vi "Keithley 2182 Edit Settings.vi"(8 "error in":errorcluster, 11 "Instrument parameters in":T1) -> (0 "error out":errorcluster, 3 "Instrument parameters out":T1)   [LabVIEW 2025]
doc: "Sets a reference for the specified measurement and reads a single Rel'd Measurement."
uses:
  Keithley 2182.lvlib
panel:
  in  "Check measurement":bool
  in  "Boolean 2":bool
  in  "Boolean":bool
  out "error out":errorcluster
  in  "stop":bool
  in  "Voltage Resolution (8)":i32=8
  in  "Range Value (0)":dbl=10.0
  in  "Auto Range (T: Enable)":bool=TRUE
  out "Measurement":dbl
  out "Measurement Metadata":T2
  in  "Measurement (0: Voltage Channel 1)":i32(ring) items=["Voltage Channel 1", "Voltage Channel 2", "Temperature Channel 1", "Temperature Channel 2"]
  in  "Integration Rate Units (0: Line Cycles)":i32(ring) items=["Line Cycles", "Seconds"]
  in  "Integration Rate (5)":dbl=5.0
  # "Settings for Keithley 2182 ..."
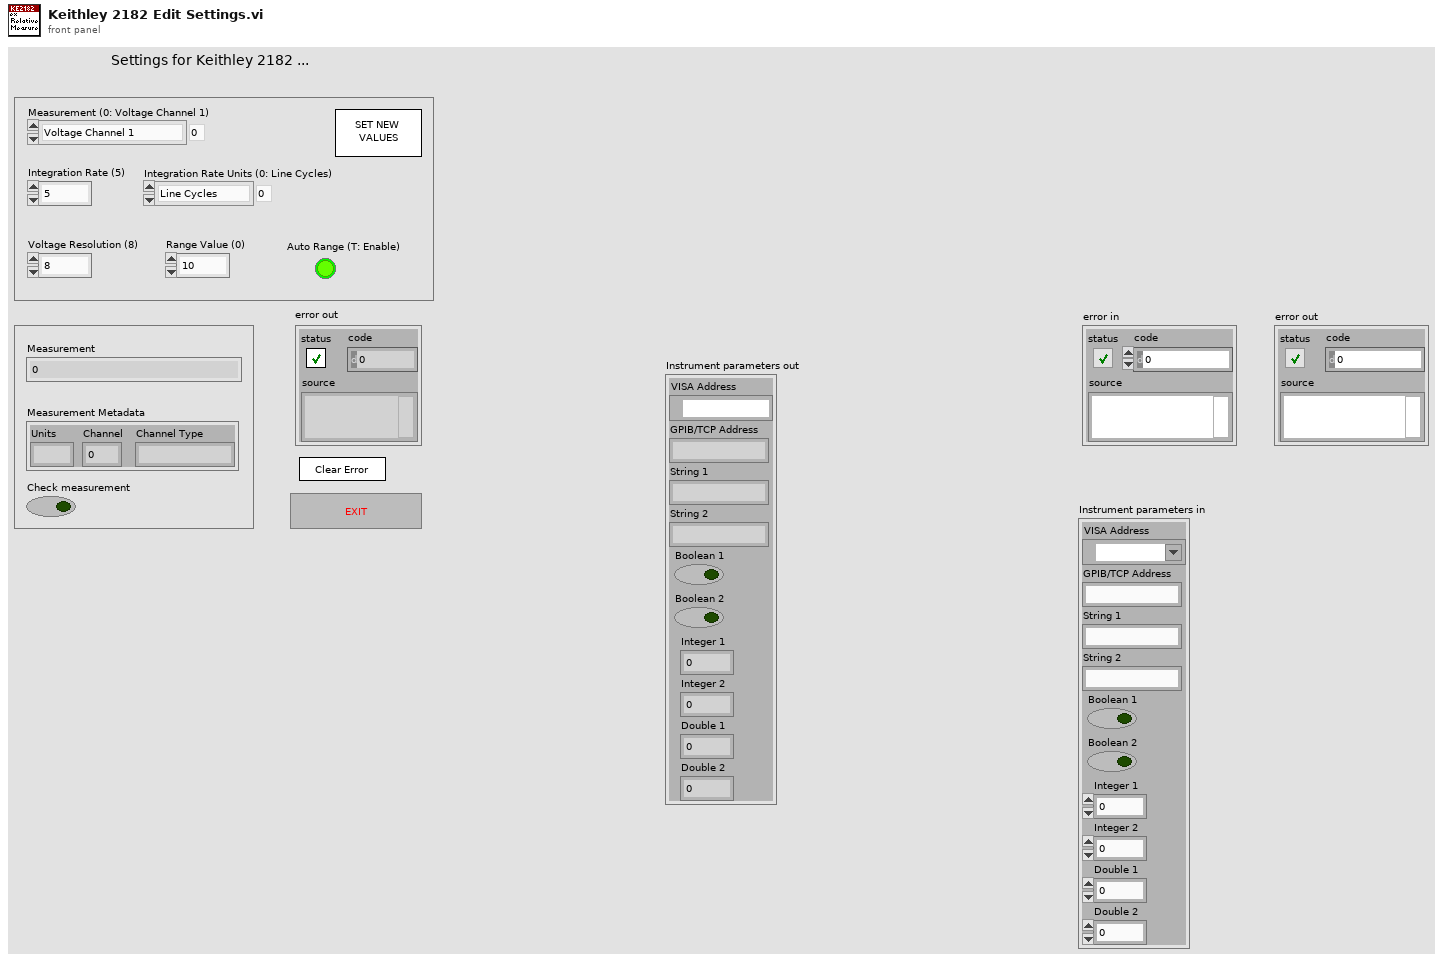
[diagram p1: front panel]
types:
  T1 = cluster{"VISA Address":refnum<visa-resource-name>, "GPIB/TCP Address":string, "String 1":string, "String 2":string, "Boolean 1":bool, "Boolean 2":bool, "Integer 1":i32, "Integer 2":i32, "Double 1":dbl, "Double 2":dbl}
  T2 = cluster{"Units":string, "Channel":i32, "Channel Type":string}
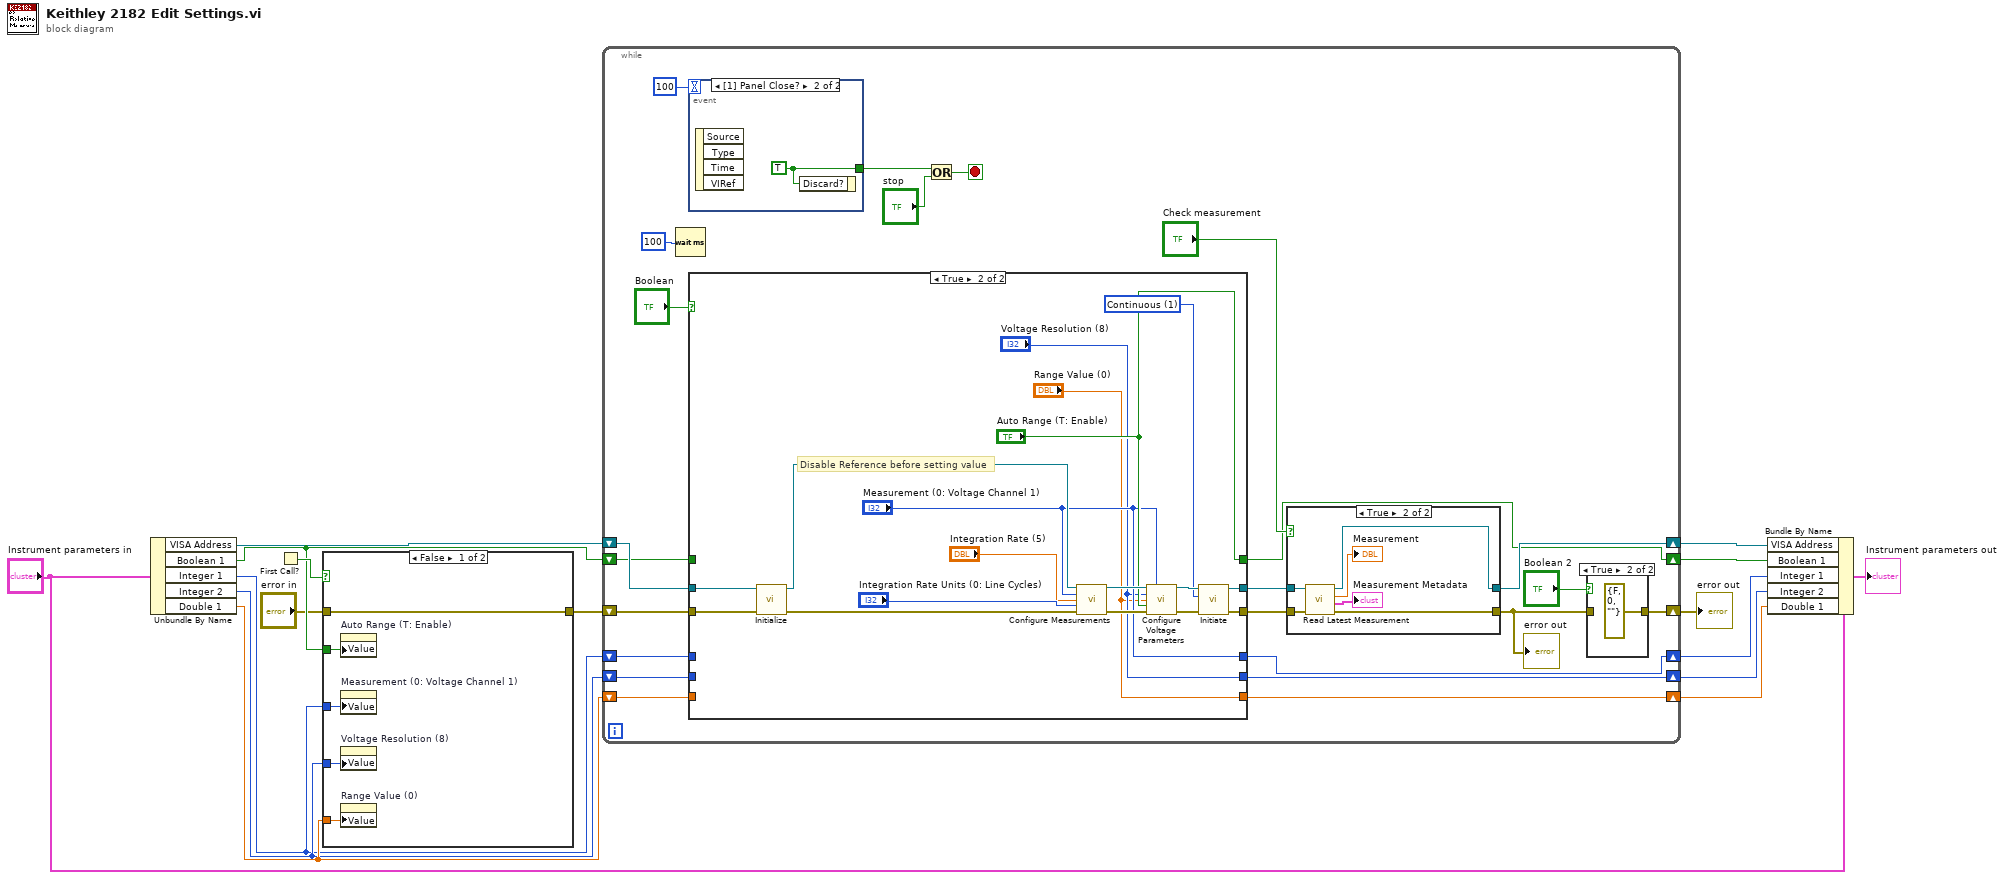
[diagram p0: block diagram]
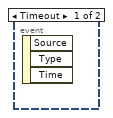
[diagram p6: hidden frame]
diagram:
  n1 = Unbundle By Name("Instrument parameters in") -> ("VISA Address"=w15:refnum<visa-resource-name>, "Boolean 1"=w4:bool, "Integer 1"=w3:i32, "Integer 2"=w5:i32, "Double 1"=w6:dbl)
  n2 = First Call?() -> (First Call?: T/F=w7:bool)
  n3 = case shown="False" w7 {
    tunnel: w6 -> [w21 _]
    tunnel: w5 -> [w20 _]
    tunnel: w4 -> [w18 _]
    tunnel: w3 -> [w19 _]
    tunnel: [w17 w22] -> w2
    tunnel: "error in" -> [w17 w22]
    frame False {
      n4 = property on="Auto Range (T: Enable)" class="Bool (strict)"("Value"=w18) -> ()  [unwired: 2 in, 2 out]
      n5 = property on="Measurement (0: Voltage Channel 1)" class="Ring (strict)"("Value"=w19) -> ()  [unwired: 2 in, 2 out]
      n6 = property on="Voltage Resolution (8)" class="DigNum (strict)"("Value"=w20) -> ()  [unwired: 2 in, 2 out]
      n7 = property on="Range Value (0)" class="DigNum (strict)"("Value"=w21) -> ()  [unwired: 2 in, 2 out]
    }
    frame True {
    }
  }
  n8 = while {
    shift-right: [w41] -> w13
    shift-left: w15 -> [w42]
    shift-right: [w34] -> w16
    shift-left: w2 -> [w40]
    shift-right: [w30] -> w11
    shift-left: w4 -> [w29]
    shift-right: [w28] -> w10
    shift-left: w3 -> [w27]
    shift-right: [w26] -> w9
    shift-left: w5 -> [w25]
    shift-right: [w23] -> w8
    shift-left: w6 -> [w24]
    stop <- w37 stop-if-true
    n9 = Wait (ms)(milliseconds to wait=u32 100) -> ()  [unwired: 1 out]
    n10 = event shown="[1] Panel Close?" {
      selector: _ -> [_ _]
      dyn-events: _ -> [_ _]
      timeout: 100 -> [_ _]
      tunnel: [_ w79] -> w39
      event Timeout {
        n11 = event-data() -> ()  [unwired: 1 in, 3 out]
      }
      event Panel Close? {
        w79 = TRUE ("Discard?")
        n12 = event-data() -> ()  [unwired: 1 in, 4 out]
        n13 = event-data("Discard?"=w79) -> ()  [unwired: 1 in, 1 out]
      }
    }
    n14 = case shown="True" "Boolean" {
      tunnel: [w60 w70] -> w45
      tunnel: [w61 w69] -> w44
      tunnel: w42 -> [w61 w67]
      tunnel: w40 -> [w60 w66]
      tunnel: [w59 "Auto Range (T: Enable)"] -> w30
      tunnel: w29 -> [w59 _]
      tunnel: [w58 "Measurement (0: Voltage Channel 1)"] -> w28
      tunnel: w27 -> [w58 _]
      tunnel: [w57 "Voltage Resolution (8)"] -> w26
      tunnel: w25 -> [w57 _]
      tunnel: [w56 "Range Value (0)"] -> w23
      tunnel: w24 -> [w56 _]
      frame False {
      }
      frame True {
        w68 = 1 items=["Immediate", "Continuous"] ("Initiate Type (0: Immediate)")
        # "Disable Reference before setting value"
        n15 = call "Initialize.vi"("error in (no error)"=w66, "VISA resource name"=w67) -> ("error out"=w78:errorcluster, "VISA resource name out"=w77:refnum<visa-resource-name>)  [unwired: 8 in]
        n16 = call "Configure Measurements.vi"("VISA resource name"=w77, "Measurement (0: Voltage Channel 1)"="Measurement (0: Voltage Channel 1)", "Integration Rate (5)"="Integration Rate (5)", "Integration Rate Units (0: Line Cycles)"="Integration Rate Units (0: Line Cycles)", "error in (no error)"=w78) -> ("VISA resource name out"=w73:refnum<visa-resource-name>, "error out"=w74:errorcluster)  [unwired: 9 in]
        n17 = call "Configure Voltage Parameters.vi"("VISA resource name"=w73, "Measurement (1: Voltage Channel 1)"="Measurement (0: Voltage Channel 1)", "Voltage Resolution (8)"="Voltage Resolution (8)", "Range Value (12)"="Range Value (0)", "Autorange (T: Enable)"="Auto Range (T: Enable)", "error in (no error)"=w74) -> ("VISA resource name out"=w71:refnum<visa-resource-name>, "error out"=w72:errorcluster)  [unwired: 8 in]
        n18 = call "Initiate.vi"("error in (no error)"=w72, "Initiate Type (0: Immediate)"=w68, "VISA resource name"=w71) -> ("error out"=w70:errorcluster, "VISA resource name out"=w69:refnum<visa-resource-name>)  [unwired: 7 in]
      }
    }
    n19 = Or(x=w39, y="stop") -> (x .or. y?=w37:bool)
    n20 = case shown="True" "Check measurement" {
      tunnel: w45 -> [w46 w53]
      tunnel: w44 -> [w47 w52]
      tunnel: [w47 w51] -> w41
      tunnel: [w46 w50] -> w33
      frame False {
      }
      frame True {
        n21 = call "Read Latest Measurement.vi"("error in (no error)"=w53, "VISA resource name"=w52) -> ("error out"=w50:errorcluster, "Measurement Metadata"=→"Measurement Metadata":T2, "Measurement"=→"Measurement":dbl, "VISA resource name out"=w51:refnum<visa-resource-name>)  [unwired: 6 in]
      }
    }
    "error out" <- w33
    n22 = case shown="True" "Boolean 2" {
      tunnel: [w54 errorcluster {"status"=FALSE, "code"=0, "source"=""} ("error out")] -> w34
      tunnel: w33 -> [w54 _]
      frame False {
      }
      frame True {
      }
    }
  }
  "error out" <- w16
  n23 = Bundle By Name(cluster="Instrument parameters in", "VISA Address"=w13, "Boolean 1"=w11, "Integer 1"=w10, "Integer 2"=w9, "Double 1"=w8) -> (→"Instrument parameters out":T1)
